vi "Parameter Save Test.vi"() -> ()   [LabVIEW 2020]
uses:
  epl-vi-lib/Signal Synthesis VIs/4th Generation/Controls/SignalManager/SignalManager.xctl
  epl-vi-lib/Signal Synthesis VIs/4th Generation/Classes/SignalManager/SignalManager.lvclass
  Classes/Parameters/Parameters.lvclass
  Classes/Parameters/Parameters.lvclass/Parameters.ctl
  Classes/State/State.lvclass/State.ctl
  Classes/Parameters/Read Flowchart.vi
  Classes/State/Read SigMan.vi
  Classes/State/State.lvclass
panel:
  in  "SignalManager":refnum<class "SignalManager.lvclass">(xcontrol)
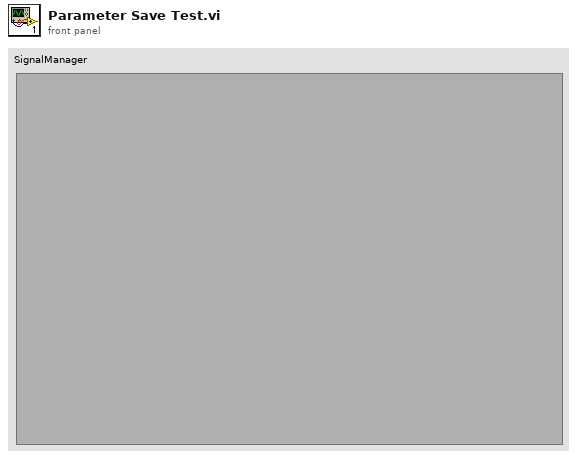
[diagram p1: front panel]
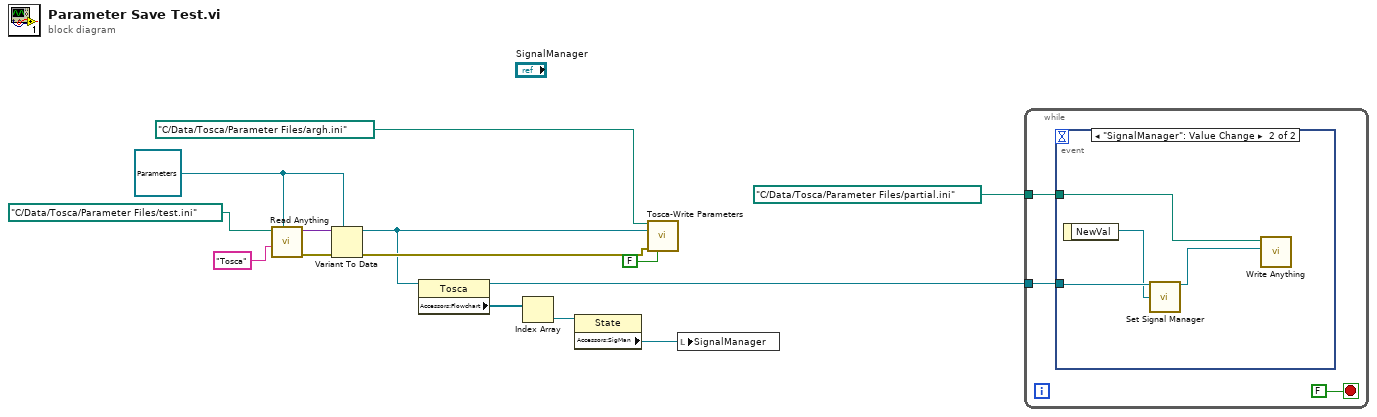
[diagram p0: block diagram]
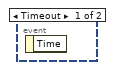
[diagram p2: hidden frame]
diagram:
  w12 = refnum<class "Parameters.lvclass"> refnum ("Tosca")
  n1 = call "Read Anything.vi"("Type of Anything"=w12, "Section Name (Name of \"Type of Anything\")"="Tosca" ("Section Name (Name of \"Anything\")"), "Path (dialog)"=path "C:/Data/Tosca/Parameter Files/test.ini") -> ("Error Out"=w11:errorcluster, "Anything"=w13:variant)  [unwired: 6 in, 1 out]
  n2 = Variant To Data(error in=w11, type=w12, Variant=w13) -> (data=w6:refnum<class "Parameters.lvclass">, error out=w9:errorcluster)
  n3 = property class="Tosca"(reference=w6) -> (reference out=w1:refnum<class "Parameters.lvclass">, "Accessors:Flowchart"=w5:refnum<class "State.lvclass">[])  [unwired: 1 in, 1 out]
  n4 = Index Array(array=w5) -> (element=w4:refnum<class "State.lvclass">)  [unwired: 1 in]
  n5 = property class="State"(reference=w4) -> ("Accessors:SigMan"=w2:refnum<class "SignalManager.lvclass">)  [unwired: 1 in, 2 out]
  n6 = call "Tosca-Write Parameters.vi"("Path in"=path "C:/Data/Tosca/Parameter Files/argh.ini" ("Path (dialog)"), "Tosca"=w6, "error in (no error)"=w9, "Prompt (T)"=FALSE) -> ()  [unwired: 9 in, 3 out]
  n7 = local write "SignalManager"(w2) -> ()
  n8 = while {
    tunnel: path "C:/Data/Tosca/Parameter Files/partial.ini" ("Path (dialog)") -> [w16]
    tunnel: w1 -> [w15]
    stop <- FALSE stop-if-true
    n9 = event shown="[1] \"SignalManager\": Value Change" {
      selector: _ -> [_ _]
      dyn-events: _ -> [_ _]
      timeout: _ -> [_ _]
      tunnel: w16 -> [_ w21]
      tunnel: w15 -> [_ w20]
      event Timeout {
        n10 = event-data() -> ()  [unwired: 1 in, 1 out]
      }
      event "SignalManager": Value Change {
        n11 = event-data() -> ("NewVal"=w19:refnum<class "SignalManager.lvclass">)  [unwired: 1 in]
        n12 = call "Set Signal Manager.vi"("Tosca in"=w20, "SigMan"=w19) -> ("Tosca out"=w18:refnum<class "Parameters.lvclass">)  [unwired: 12 in, 1 out]
        n13 = call "Write Anything.vi"("Anything"=w18, "Path (dialog)"=w21) -> ()  [unwired: 8 in, 2 out]
      }
    }
  }
